vi "Obtain cycle time.vi"() -> (1 "Funct Acq Cycle time (sec)":dbl, 2 "Funct Acq cycle length (us)":dbl)   [LabVIEW 2013]
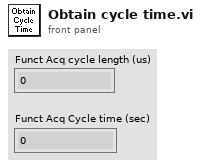
[diagram p1: front panel]
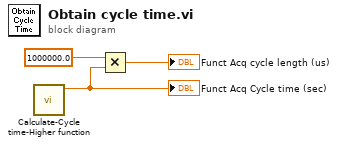
[diagram p0: block diagram]
diagram:
  n1 = call "Calculate-Cycle time-Higher function.vi"() -> ("Cycle Time (s)"=w3:dbl)  [unwired: 11 in]
  "Funct Acq Cycle time (sec)" <- w3
  n2 = Multiply(x=1000000.0, y=w3) -> (x*y=→"Funct Acq cycle length (us)":dbl)
